vi "Concatenation_2strings.vi"() -> ()   [LabVIEW 2020]
panel:
  out "Chaîne Result":string
  in  "chaine2":string
  in  "chaine1":string
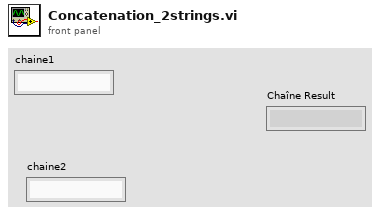
[diagram p1: front panel]
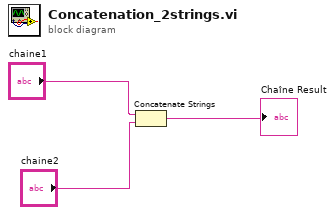
[diagram p0: block diagram]
diagram:
  n1 = Concatenate Strings("chaine1", "chaine2") -> (→"Chaîne Result":string)
